vi "GreyRightRing.vi"(8 "error in (no error)":errorcluster, 11 "MAUI in":refnum<class "MAUI.lvclass">) -> (0 "error out":errorcluster, 3 "MAUI out":refnum<class "MAUI.lvclass">)   [LabVIEW 2016, in "MAUI.lvclass"]
uses:
  MAUI.lvclass
  MAUI.lvclass/MAUI.ctl
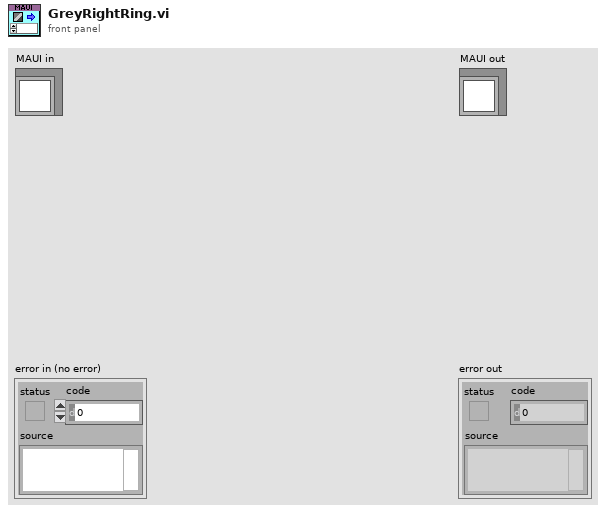
[diagram p1: front panel]
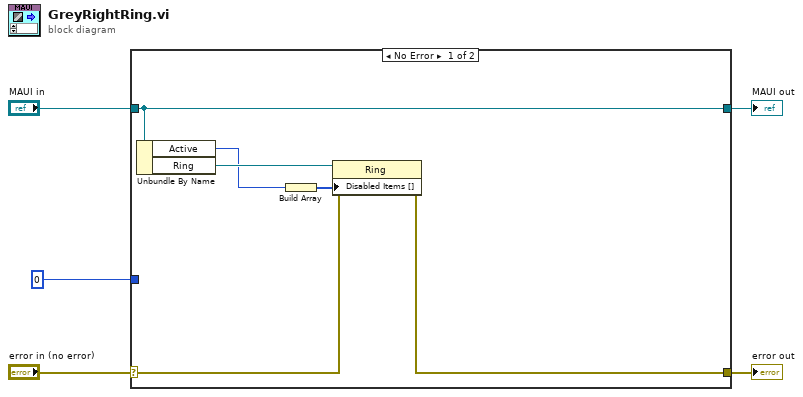
[diagram p0: block diagram]
diagram:
  n1 = case shown="No Error" "error in (no error)" {
    selector: "error in (no error)" -> [w8 w13]
    tunnel: [w7 w13] -> w4
    tunnel: [w11 w12] -> w2
    tunnel: "MAUI in" -> [w11 w12]
    tunnel: 0 -> [_ _]
    frame No Error {
      n2 = Unbundle By Name(w11) -> ("Active"=w6:i32, "Ring"=w10:refnum<vi>)
      n3 = Build Array(w6) -> (w9:i32[])
      n4 = property class="Ring"(reference=w10, error in=w8, "Disabled Items []"=w9) -> (error out=w7:errorcluster)  [unwired: 1 out]
    }
    frame Error {
    }
  }
  "error out" <- w4
  "MAUI out" <- w2
